vi "Set Rate and Buffer.vi"(8 "error in (no error)":errorcluster, 11 "DAQ Task in":refnum<class "DAQ Task.lvclass">) -> (0 "error out":errorcluster, 3 "DAQ Task out":refnum<class "DAQ Task.lvclass">)   [LabVIEW 2012, in "Data Acquisition.lvlib" / "DAQ Task.lvclass"]
uses:
  DAQ Task.lvclass
  DAQ Task.lvclass/DAQ Task.ctl
  <vilib>/DAQmx/configure/timing.llb/DAQmx Timing (Sample Clock).vi
  <resource>/objmgr/daqmx.rc
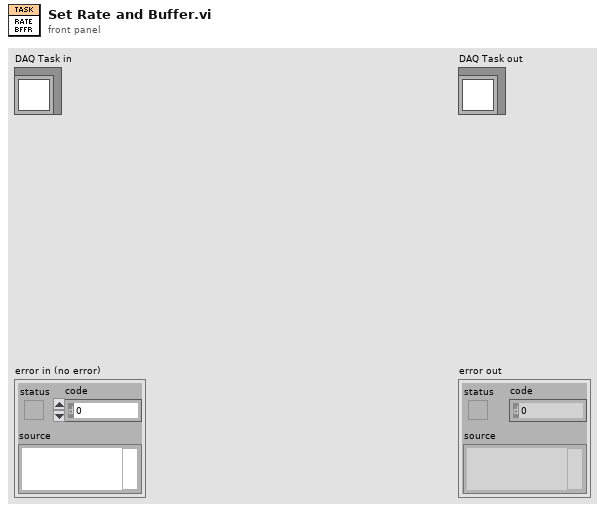
[diagram p1: front panel]
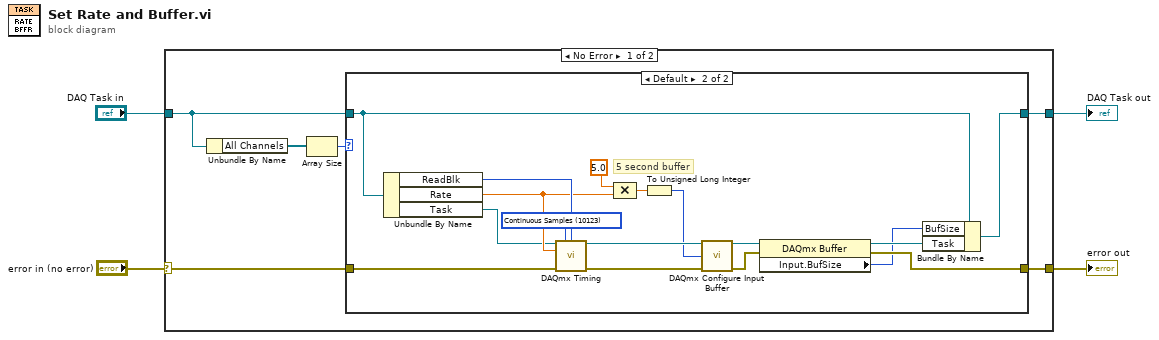
[diagram p0: block diagram]
diagram:
  n1 = case shown="No Error" "error in (no error)" {
    selector: "error in (no error)" -> [w10 w31]
    tunnel: [w8 w31] -> w4
    tunnel: [w9 w30] -> w1
    tunnel: "DAQ Task in" -> [w7 w30]
    frame No Error {
      n2 = Unbundle By Name(w7) -> ("All Channels"=w6:refnum<class "Channel.lvclass">[])
      n3 = Array Size(array=w6) -> (size(s)=w5:i32)
      n4 = case shown="Default" w5 {
        tunnel: w10 -> [w11 w29]
        tunnel: [w12 w28] -> w9
        tunnel: [w11 w14] -> w8
        tunnel: w7 -> [w12 w18]
        frame 0 {
        }
        frame Default {
          w27 = 10123 items=["Finite Samples"=10178, "Continuous Samples"=10123, "Hardware Timed Single Point"=12522] ("sample mode")
          # "5 second buffer"
          n5 = Unbundle By Name(w18) -> ("ReadBlk"=w24:i32, "Rate"=w21:dbl, "Task"=w19:refnum<k21>)
          n6 = call-poly <vilib>:"DAQmx Timing.vi"("task/channels in"=w19, "sample mode"=w27, "samples per channel"=w24, "rate"=w21, "error in"=w29) -> ("task out"=w26:refnum<k21>, "error out"=w25:errorcluster)  [unwired: 9 in]
          n7 = Compound Arithmetic op=MULTIPLY(5.0 ("Rate"), w21) -> (w23:dbl)
          n8 = To Unsigned Long Integer(number=w23) -> (unsigned 32bit integer=w22:u32)
          n9 = call <vilib>:"DAQmx Configure Input Buffer.vi"("task/channels in"=w26, "buffer size (in samples per channel)"=w22, "error in"=w25) -> ("task out"=w17:refnum<k21>, "error out"=w15:errorcluster)  [unwired: 11 in]
          n10 = property class="DAQmx Buffer"(reference=w17, error in=w15) -> (reference out=w16:refnum<k21>, error out=w14:errorcluster, "Input.BufSize"=w13:u32)
          n11 = Bundle By Name(cluster=w18, "BufSize"=w13, "Task"=w16) -> (w28:refnum<class "DAQ Task.lvclass">)
        }
      }
    }
    frame Error {
    }
  }
  "error out" <- w4
  "DAQ Task out" <- w1
